vi "GPIB_autodetect.vi"(8 "error in (no error)":errorcluster, 9 "Verify GPIB address":bool, 10 "Instrument GPIB address in":string, 11 "KE487 in":refnum<class "KE487.lvclass">) -> (0 "error out":errorcluster, 2 "Instrument GPIB address":string, 3 "KE487 out":refnum<class "KE487.lvclass">)   [LabVIEW 2018, in "KE487.lvclass"]
uses:
  KE487.lvclass
  InstrControl.lvclass
panel:
  out "GPIB addresses found":string[](array[string])
  out "IDN? responses":string[](array[string])
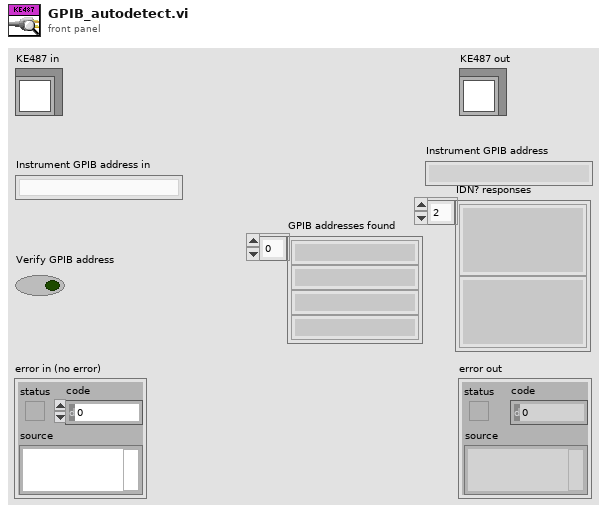
[diagram p1: front panel]
types:
  T1 = cluster{"error":bool, "code":i32, "source":string}
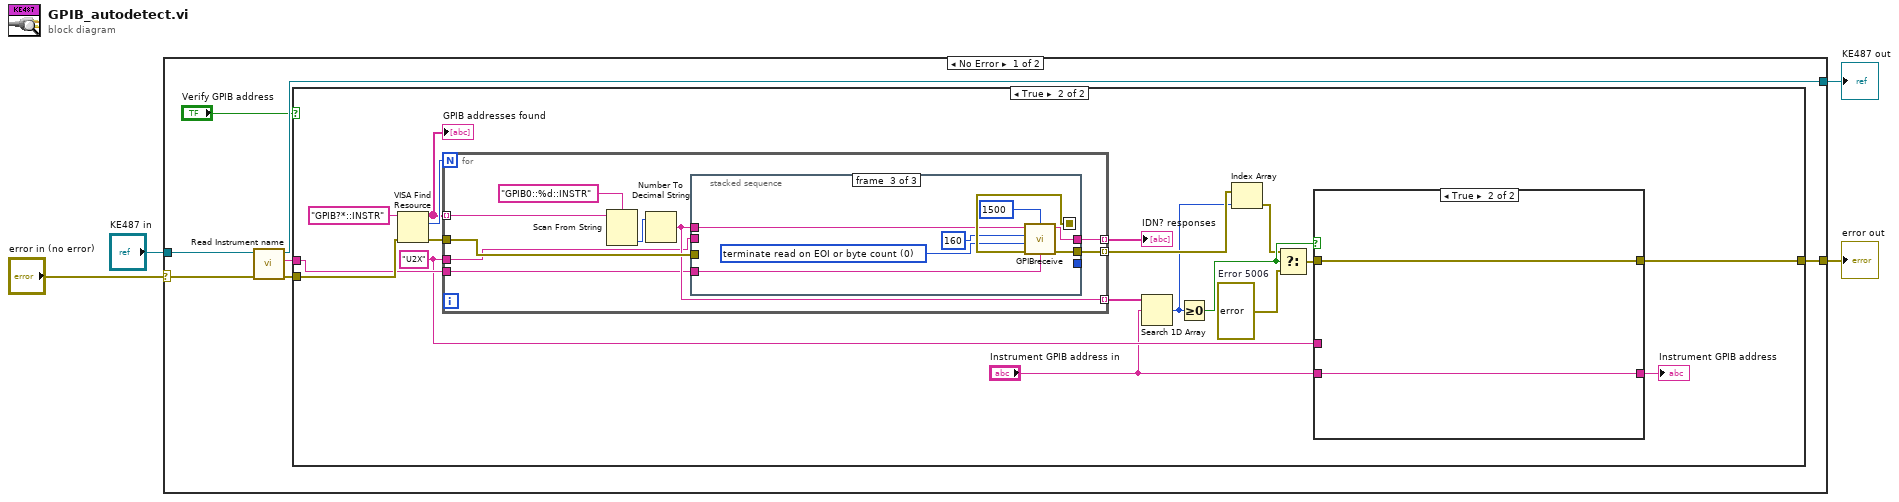
[diagram p0: block diagram]
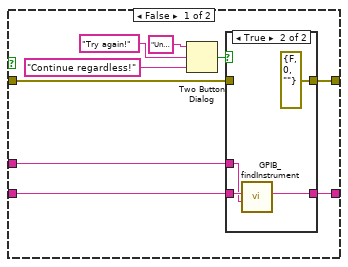
[diagram p3: hidden frame]
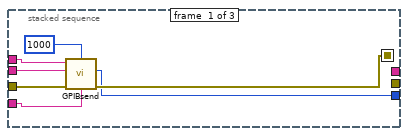
[diagram p5: hidden frame]
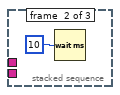
[diagram p6: hidden frame]
diagram:
  n1 = case shown="No Error" "error in (no error)" {
    selector: "error in (no error)" -> [w10 w74]
    tunnel: [w7 w74] -> w1
    tunnel: [w9 w73] -> w4
    tunnel: "KE487 in" -> [w11 w73]
    frame No Error {
      n2 = call-dynamic "Read Instrument name.vi"("error in (no error)"=w10, "InstControl in"=w11) -> ("error out"=w8:errorcluster, "Instrument name"=w6:string, "InstControl out"=w9:refnum<class "KE487.lvclass">)  [unwired: 7 in]
      n3 = case shown="True" "Verify GPIB address" {
        tunnel: w8 -> [w12 w25]
        tunnel: [w12 w20] -> w7
        tunnel: w6 -> [_ w19]
        frame False {
        }
        frame True {
          w17 = "U2X"
          w30 = errorcluster {"status"=FALSE, "code"=5005, "source"="Unable to find specified instrument.  Please make sure the it is connected to your system and switched on."}  # Error 5006
          n4 = VISA Find Resource(8:w25, 11:"GPIB?*::INSTR" ("expression (\"\")")) -> (0:w29:errorcluster, 2:w28:u32, 3:w27:string[])  [unwired: 1 in]
          "GPIB addresses found" <- w27
          n5 = for {
            N: w28 -> [_]
            tunnel: w27 -> [w54] mode=indexing
            tunnel: w29 -> [w56]
            tunnel: [w55] -> w15 mode=indexing
            tunnel: [w50] -> w23 mode=indexing
            tunnel: w19 -> [w49]
            tunnel: [w51] -> w26 mode=indexing
            tunnel: w17 -> [w48]
            n6 = Scan From String(format string="GPIB0::%d::INSTR" ("expression (\"\")"), input string=w54) -> (output 1=w52:i32)  [unwired: 3 in, 3 out]
            n7 = Number To Decimal String(number=w52) -> (decimal integer string=w50:string)  [unwired: 1 in]
            n8 = stacked-sequence {
              seq-local: [w61 _ _] -> [_ _ w71]
              tunnel: w50 -> [w63 _ w70]
              tunnel: w56 -> [w62 _ _]
              tunnel: [_ _ w72] -> w55
              tunnel: [_ _ w67] -> w51
              tunnel: w49 -> [w59 _ w68]
              tunnel: w48 -> [w58 _ _]
              tunnel: [w57 _ _] -> _
              frame #0 {
                n9 = call "GPIBsend.vi"("timeout ms"=u32 1000, "address string"=w63, "write buffer"=w58, "source"=w59, "error in"=w62) -> ("byte count"=w57:i32, "error out"=w61:errorcluster)  [unwired: 2 in, 1 out]
              }
              frame #1 {
                n10 = Wait (ms)(milliseconds to wait=10) -> ()  [unwired: 1 out]
              }
              frame #2 {
                w66 = 0 items=["terminate read on EOI or byte count", "terminate read on EOI, byte count, or CR", "terminate read on EOI, byte count, or LF"] ("read mode")
                n11 = call "GPIBreceive.vi"("timeout ms"=u32 1500, "address string"=w70, "byte count"=160, "source"=w68, "read mode"=w66, "error in"=w71) -> ("read buffer"=w67:string, "error out"=w72:T1)  [unwired: 1 in, 1 out]
              }
            }
          }
          "IDN? responses" <- w26
          n12 = Search 1D Array(1D array=w23, element="Instrument GPIB address in") -> (index of element=w14:i32)  [unwired: 1 in]
          n13 = Greater Or Equal To 0?(x=w14) -> (x >= 0?=w22:bool)
          n14 = Index Array(array=w15, index=w14) -> (element=w13:T1)
          n15 = Select(t=w13, s=w22, f=w30) -> (s? t:f=w21:errorcluster)
          n16 = case shown="True" w22 {
            tunnel: "Instrument GPIB address in" -> [w35 w47]
            tunnel: [w34 w47] -> w18
            tunnel: w21 -> [w33 w46]
            tunnel: [w32 w46] -> w20
            tunnel: w17 -> [w31 _]
            frame False {
              n17 = Two Button Dialog(message="Unable to find specified instrument.  Please make sure the it is connected to your system and switched on." ("source"), 1:"Continue regardless!", 2:"Try again!") -> (T button?=w36:bool)
              n18 = case shown="True" w36 {
                tunnel: w35 -> [w41 w45]
                tunnel: [w41 w44] -> w34
                tunnel: w33 -> [w40 _]
                tunnel: [w40 errorcluster {"status"=FALSE, "code"=0, "source"=""} ("error constant")] -> w32
                tunnel: w31 -> [_ w42]
                frame False {
                }
                frame True {
                  n19 = call "GPIB_findInstrument.vi"("ID command"=w42, "revised GPIB address"=w45) -> ("revised GPIB address OUT"=w44:string)  [unwired: 9 in]
                }
              }
            }
            frame True {
            }
          }
          "Instrument GPIB address" <- w18
        }
      }
    }
    frame Error {
    }
  }
  "error out" <- w1
  "KE487 out" <- w4
